vi "HFRR ADV v013 new software.vi"() -> ()   [LabVIEW 2025] (continued)
                n4035 = VISA Write(VISA resource name=w5224, write buffer=w5220, error in (no error)=w5223) -> (VISA resource name out=w5222:refnum<visa-resource-name>, error out=w5221:errorcluster)  [unwired: 1 out]
                n4036 = local write item#-1(FALSE ("WRITE")) -> ()
              }
            }
          }
          frame Error {
            w5312 = u16 10 items=["1.0"=10, "1.5"=15, "2.0"=20] ("stop bits (10: 1 bit)")
            n4037 = Wait (ms)(milliseconds to wait=u32 20) -> ()  [unwired: 1 out]
            n4038 = VISA Close(VISA resource name=w5314, error in (no error)=w5320) -> (error out=w5319:errorcluster)
            n4039 = call <vilib>:"Clear Errors.vi"("error in (no error)"=w5319) -> ("error out"=w5318:errorcluster)  [unwired: 5 in, 1 out]
            n4040 = call-poly "VISA Configure Serial Port"("timeout (10sec)"=u32 200, "Enable Termination\nChar (T)"=TRUE ("Enable Termination\nChar (T)"), "baud rate (9600)"=u32 921600, "error in (no error)"=w5318, "stop bits (10: 1 bit)"=w5312) -> ("VISA resource name"=w5310:refnum<visa-resource-name>, "VISA resource name out"=w5322:refnum<visa-resource-name>, "error out"=w5321:errorcluster)  [unwired: 8 in]
          }
        }
        n4041 = local read "Quit"() -> (w5162:bool)
      }
      n4042 = VISA Close(VISA resource name=w5157, error in (no error)=w5158) -> (error out=w5156:errorcluster)
      n4043 = call <vilib>:"Clear Errors.vi"("error in (no error)"=w5156) -> ()  [unwired: 5 in, 2 out]
    }
    frame Enabled {
    }
  }
  n4044 = disable-structure shown="Disabled" {
    disable-tunnel: _ -> [w5327 _]
    frame Disabled {
      n4045 = while {
        tunnel: [w5334] -> _
        shift-right: [w5331] -> w5324
        shift-left: _ -> [w5333]
        shift-right: [w5332] -> w5325
        shift-left: errorcluster {"status"=TRUE, "code"=0, "source"="Init"} ("error out") -> [w5330]
        tunnel: w5327 -> [_]
        i -> [w5334]
        stop <- w5328 stop-if-true
        n4046 = flat-sequence {
          tunnel: w5330 -> [w5425]
          tunnel: [w5425] -> w5329
          frame #0 {
            n4047 = Wait (ms)(milliseconds to wait=u32 50) -> ()  [unwired: 1 out]
          }
        }
        n4048 = case shown="No Error" w5329 {
          selector: w5329 -> [w5375 w5418]
          tunnel: w5333 -> [w5374 w5417]
          tunnel: [w5341 w5408] -> w5332
          tunnel: [w5342 w5416] -> w5331
          frame No Error {
            w5368 = T32 {"Mode"=enum."RTU", "Slave Address"=1} ("Serial Parameters")
            n4049 = call-poly <vilib>:"MB Serial Master Query (poly).vi"("VISA resource name"=w5374, "Starting Address"=i16 1000, "Quantity"=u16 1, "Timeout"=u32 1000, "error in"=w5375, "Serial Parameters"=w5368) -> ("VISA resource name out"=w5369:refnum<visa-resource-name>, "Input Registers"=w5371:u16[], "error out"=w5367:errorcluster)  [unwired: 10 in, 1 out]
            n4050 = Random Number (0-1)() -> (number: 0 to 1=w5356:dbl)
            n4051 = Index Array(array=w5371, index=0) -> (element=w5366:u16)
            n4052 = Subtract(x=w5356, y=0.5) -> (x-y=w5355:dbl)
            n4053 = Divide(x=w5366, y=10 ("index")) -> (x/y=w5360:dbl)
            n4054 = Multiply(x=w5355, y=0.5) -> (x*y=w5354:dbl)
            n4055 = Add(x=w5360, y=w5354) -> (x+y=w5359:dbl)
            n4056 = local read "Amb temp"() -> (w5343:dbl)
            n4057 = Multiply(x=w5359, y=0.2) -> (x*y=w5363:dbl)
            n4058 = Multiply(x=w5343, y=0.8) -> (x*y=w5361:dbl)
            n4059 = Add(x=w5363, y=w5361) -> (x+y=w5344:dbl)
            n4060 = local read "set temp old"() -> (w5338:dbl)
            n4061 = local write "Amb temp"(w5344) -> ()
            n4062 = Select(t="SetTemp 2", s="Heater", f=100.0) -> (s? t:f=w5339:dbl)
            n4063 = Not Equal?(x=w5339, y=w5338) -> (x != y?=w5337:bool)
            n4064 = case shown="True" w5337 {
              tunnel: w5369 -> [w5403 w5405]
              tunnel: [w5402 w5405] -> w5349
              tunnel: w5367 -> [w5401 w5404]
              tunnel: [w5400 w5404] -> w5347
              tunnel: w5339 -> [w5395 _]
              tunnel: w5368 -> [w5397 w5406]
              tunnel: [w5397 w5406] -> w5350
              frame True {
                n4065 = Multiply(x=w5395, y=10 ("index")) -> (x*y=w5394:dbl)
                n4066 = call-poly <vilib>:"MB Serial Master Query (poly).vi"("VISA resource name"=w5403, "Address"=u16 0, "Holding Register"=w5394, "Timeout"=u32 1000, "error in"=w5401, "Serial Parameters"=w5397) -> ("VISA resource name out"=w5402:refnum<visa-resource-name>, "error out"=w5400:errorcluster)  [unwired: 11 in, 1 out]
                "set temp old" <- w5395
              }
              frame False {
              }
            }
            n4067 = flat-sequence {
              tunnel: [w5376] -> _
              tunnel: [w5376] -> w5346
              tunnel: w5347 -> [w5376]
              frame #0 {
                n4068 = Wait (ms)(milliseconds to wait=u32 100) -> ()  [unwired: 1 out]
              }
            }
            n4069 = call "Elapsed Time12"("Time Target (s)"=2.0, "Auto Reset"=TRUE) -> ("Time has Elapsed"=w5351:bool)  [unwired: 10 in, 7 out]
            n4070 = case shown="True" w5351 {
              tunnel: w5350 -> [w5380 w5393]
              tunnel: [w5380 w5393] -> _
              tunnel: [w5379 w5391] -> w5342
              tunnel: w5349 -> [w5379 w5392]
              tunnel: [w5378 w5389] -> w5341
              tunnel: w5346 -> [w5378 w5390]
              frame False {
              }
              frame True {
                n4071 = call-poly <vilib>:"MB Serial Master Query (poly).vi"("VISA resource name"=w5392, "Starting Address"=i16 1003 ("Addr"), "Quantity"=u16 1, "Timeout"=u32 1000, "error in"=w5390, "Serial Parameters"=w5393) -> ("VISA resource name out"=w5391:refnum<visa-resource-name>, "Input Registers"=w5386:u16[], "error out"=w5389:errorcluster)  [unwired: 10 in, 1 out]
                n4072 = Index Array(array=w5386, index=0) -> (element=w5385:u16)
                n4073 = Divide(x=w5385, y=u16 10) -> (x/y=w5381:dbl)
                n4074 = local write "set temp old"(w5381) -> ()
                n4075 = local write "SetTemp"(w5381) -> ()
              }
            }
            "Error Code" <- w5341
            n4076 = Unbundle(w5341) -> ("status"=→"TK4 status":bool)  [unwired: 2 out]
            "SetTemp" <- "SetTemp 2"
          }
          frame Error {
            w5420 = u16 0 items=["None", "Odd", "Even", "Mark", "Space"] ("Parity")
            w5421 = u16 0 items=["None", "XON/XOFF", "RTS/CTS", "XON/XOFF & RTS/CTS", "DTR/DSR", "XON/XOFF & DTR/DSR"] ("Flow Control")
            n4077 = VISA Clear(VISA resource name=w5417, error in (no error)=w5418) -> (VISA resource name out=w5411:refnum<visa-resource-name>, error out=w5409:errorcluster)
            n4078 = VISA Close(VISA resource name=w5411, error in (no error)=w5409) -> (error out=w5410:errorcluster)
            n4079 = call <vilib>:"Clear Errors.vi"("error in (no error)"=w5410) -> ("error out"=w5419:errorcluster)  [unwired: 5 in, 1 out]
            n4080 = Unbundle By Name(T32 {"Mode"=enum."RTU", "Slave Address"=1} ("input cluster")) -> ("Mode"=w5422:enum16{"RTU", "ASCII"})
            n4081 = call <vilib>:"MB Serial Init.vi"("Timeout"=u32 100, "Flow Control"=w5421, "Mode"=w5422, "error in (no error)"=w5419, "Parity"=w5420, "Baud Rate"=u32 9600, "VISA resource name"="Lubrication System COM Port :") -> ("error out"=w5408:errorcluster, "VISA resource name out"=w5416:refnum<visa-resource-name>)  [unwired: 3 in]
            n4082 = local write "set temp old"(0.0 ("set temp old")) -> ()
            n4083 = Unbundle(w5408) -> ("status"=w5407:bool)  [unwired: 2 out]
            n4084 = case shown="True" w5407 {
              selector: w5407 -> [_ w5424]
              frame False {
              }
              frame True {
                n4085 = local write "TK4 status"(w5424) -> ()
              }
            }
          }
        }
        n4086 = local read "Quit"() -> (w5328:bool)
      }
      n4087 = VISA Close(VISA resource name=w5324, error in (no error)=w5325) -> (error out=w5323:errorcluster)
      n4088 = call <vilib>:"Clear Errors.vi"("error in (no error)"=w5323) -> ()  [unwired: 5 in, 2 out]
    }
    frame Enabled {
    }
  }
